vi "IMAQdx Prototyping-mod.vi"() -> ()   [LabVIEW 2017]
uses:
  <vilib>/userdefined/High Color/IMAQdx.ctl
  <vilib>/vision/Avi.llb/IMAQ AVI2 Codec Path.ctl
  <vilib>/vision/driver/IMAQdx.llb/IMAQdx Buffer Number Mode.ctl
  <vilib>/vision/driver/NI_Vision_Acquisition_Software.lvlib
  <vilib>/vision/NI_Vision_Development_Module.lvlib
panel:
  out "Missed frames!":bool
  out "Buffer Number Delta":u32
  out "Skipped Buffer Count":u32
  out "Acquired Frame Rate":dbl
  out "Processed Frame Rate":dbl
  in  "Vertical Stop Button":bool
  in  "Capture video":bool
  out "Codec Names":string[](array[string])
  out "element":string
  in  "index":i32=6
  in  "AVI Path":path=path "C:/Users/Theo/Desktop/AVI compression tests"
  in  "Resolution":dbl(slide)=1.0 step=0.1 scale=0.1..1.0
  in  "Interpolation Type":u32(ring) items=["Zero Order", "Bi-Linear", "Quadratic", "Cubic Spline"]
  out "Image 2":T1(plugin-control)
  out "ms":u32 format="%.0f ms"
  out "Image":T1(plugin-control)
  in  "Session In":T2="cam0"
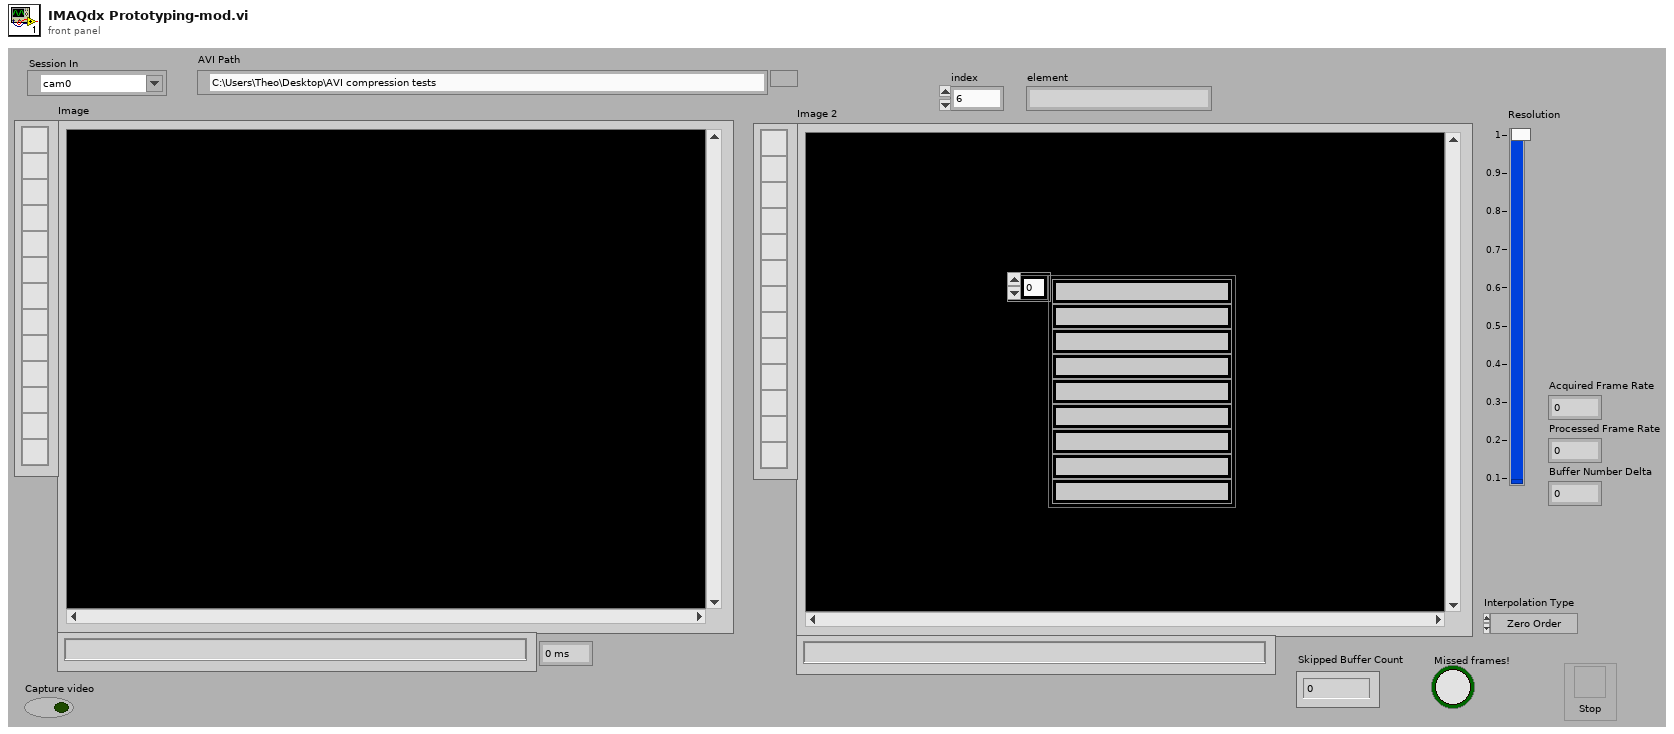
[diagram p1: front panel]
types:
  T1 = typedef "IMAQ Image.ctl" = refnum<image>
  T2 = typedef "IMAQdx.ctl" = refnum<k21>
  T3 = typedef "IMAQ AVI2 Codec Path.ctl" = u32
  T4 = typedef "Image Type" = u32
  T5 = enum16{"open", "replace", "create", "open or create", "replace or create", "replace or create with confirmation"}
  T6 = typedef "IMAQ AVI2 Refnum.ctl" = refnum<k20>
  T7 = typedef "NI_Vision_Acquisition_Software.lvlib/IMAQdx Buffer Number Mode.ctl" = enum32{"Next", "Last", "Buffer Number", "Every", "Last New"}
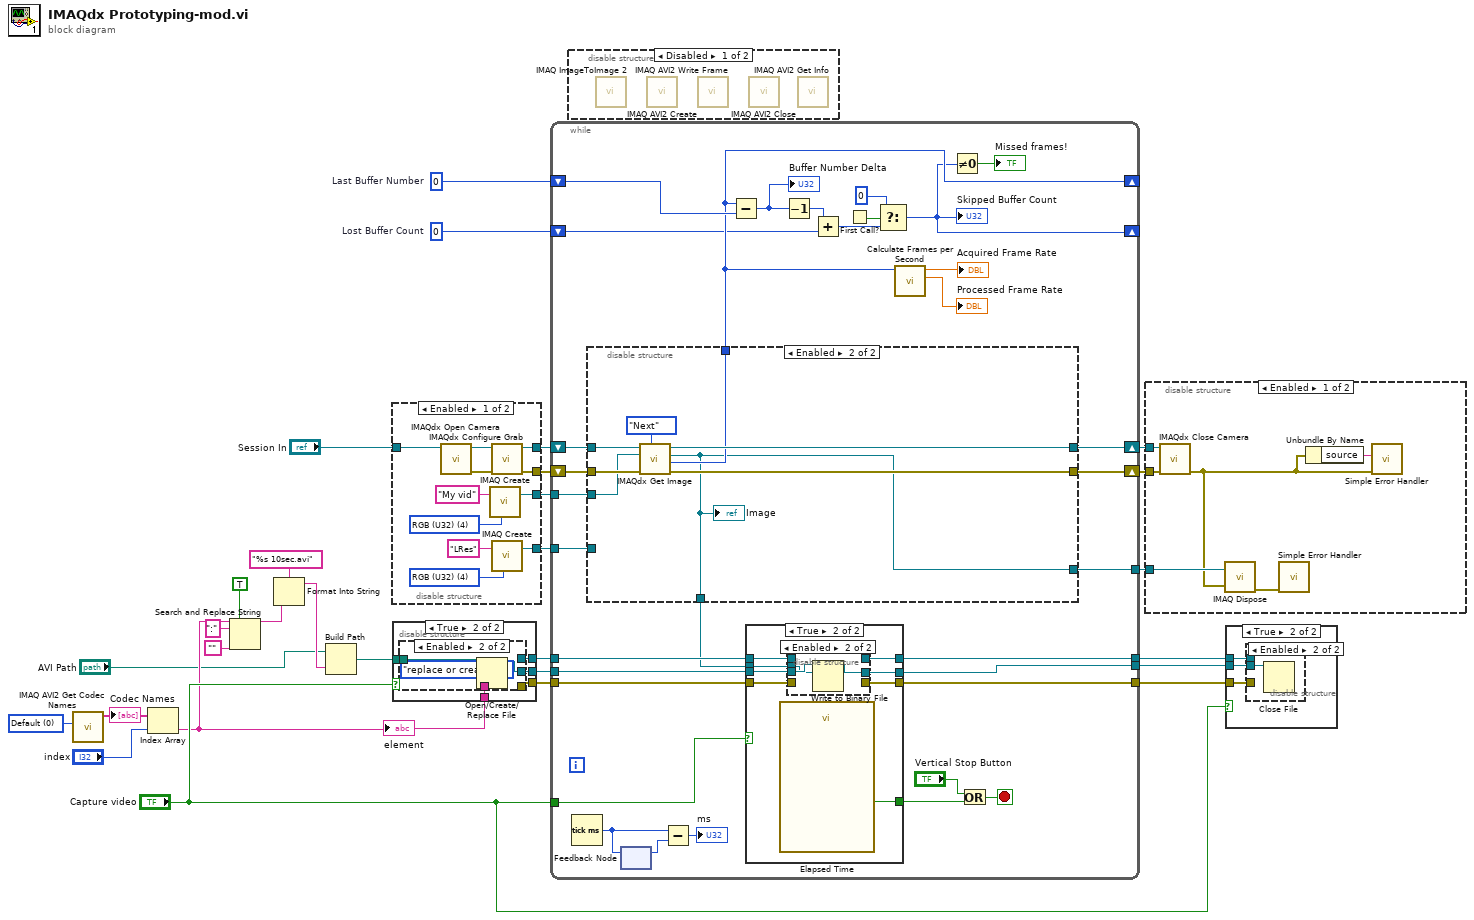
[diagram p0: block diagram]
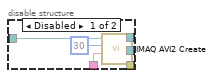
[diagram p5: hidden frame]
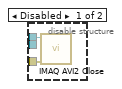
[diagram p7: hidden frame]
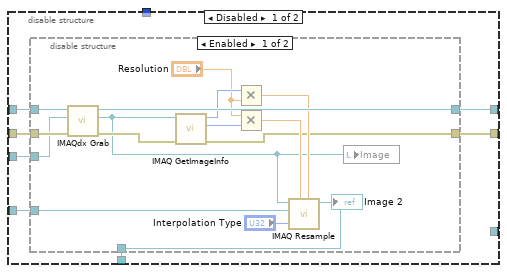
[diagram p9: hidden frame]
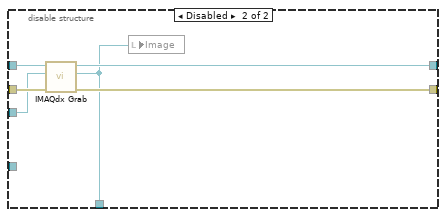
[diagram p10: hidden frame]
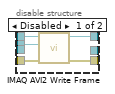
[diagram p12: hidden frame]
diagram:
  w10 = u32 0  # Lost Buffer Count
  w11 = u32 0  # Last Buffer Number
  w29 = T3 0 items=["Default", "System", "Built in Vision"] ("Codec Source")
  n1 = call "IMAQ AVI2 Get Codec Names"("Codec Source"=w29) -> ("Codec Names"=w22:string[])  [unwired: 9 in, 1 out]
  "Codec Names" <- w22
  n2 = Index Array(array=w22, index="index") -> (element=w6:string)
  "element" <- w6
  n3 = Search and Replace String(replace all?=TRUE ("replace all? (F)"), input string=w6, search string=":", replace string="" ("replace string (\"\")")) -> (result string=w7:string)  [unwired: 4 in, 3 out]
  n4 = Format Into String(format string="%s 10sec.avi", w7) -> (resulting string=w13:string)  [unwired: 2 in, 1 out]
  n5 = Build Path(base path="AVI Path", name or relative path=w13) -> (appended path=w15:path)
  n6 = disable-structure shown="Enabled" {
    disable-tunnel: [w40 _] -> w28
    disable-tunnel: [w39 _] -> w25
    disable-tunnel: [w36 _] -> w24
    disable-tunnel: [w34 _] -> w23
    disable-tunnel: "Session In" -> [w32 _]
    frame Enabled {
      w33 = T4 4 items=["Grayscale (U8)", "Grayscale (I16)", "Grayscale (SGL)", "Complex (CSG)", "RGB (U32)", "HSL (U32)", "RGB (U64)", "Grayscale (U16)"] ("Image Type")
      w37 = T4 4 items=["Grayscale (U8)", "Grayscale (I16)", "Grayscale (SGL)", "Complex (CSG)", "RGB (U32)", "HSL (U32)", "RGB (U64)", "Grayscale (U16)"] ("Image Type")
      n7 = call <vilib>:"IMAQdx Open Camera.vi"("Session In"=w32) -> ("error out"=w30:errorcluster, "Session Out"=w31:T2)  [unwired: 9 in]
      n8 = call "IMAQ Create"("Image Name"="My vid", "Image Type"=w37) -> ("New Image"=w36:T1)  [unwired: 3 in, 1 out]
      n9 = call <vilib>:"IMAQdx Configure Grab.vi"("error in"=w30, "Session In"=w31) -> ("error out"=w39:errorcluster, "Session Out"=w40:T2)  [unwired: 8 in]
      n10 = call "IMAQ Create"("Image Name"="LRes", "Image Type"=w33) -> ("New Image"=w34:T1)  [unwired: 3 in, 1 out]
    }
    frame Disabled {
    }
  }
  n11 = case shown="True" "Capture video" {
    tunnel: w15 -> [_ w45]
    tunnel: [_ w44] -> w20
    tunnel: [_ w43] -> w19
    tunnel: w6 -> [_ w42]
    tunnel: [_ w41] -> w2
    frame False {
    }
    frame True {
      n12 = disable-structure shown="Enabled" {
        disable-tunnel: w45 -> [w50 w53]
        disable-tunnel: [w48 _] -> w44
        disable-tunnel: [w47 _] -> w43
        disable-tunnel: w42 -> [w46 _]
        disable-tunnel: [_ w52] -> w41
        frame Disabled {
          n13 = call "IMAQ AVI2 Create"("Codec"=w46, "Frames Per Second"=u32 30, "AVI Path"=w50) -> ("error out"=w47:errorcluster, "AVI Refnum"=w48:T6)  [unwired: 7 in]
        }
        frame Enabled {
          n14 = Open/Create/Replace File(file path (use dialog)=w53, operation (0:open)=T5."replace or create") -> (refnum out=w52:refnum<file>)  [unwired: 4 in, 2 out]
        }
      }
    }
  }
  n15 = while {
    shift-right: [w85] -> w27
    shift-left: w28 -> [w86]
    shift-right: [w75] -> w26
    shift-left: w25 -> [w84]
    tunnel: w24 -> [w83]
    tunnel: w23 -> [w79]
    tunnel: w20 -> [w78]
    tunnel: w19 -> [w77]
    tunnel: [w76] -> w18
    tunnel: [w73] -> w17
    tunnel: "Capture video" -> [w72]
    tunnel: [w68] -> w12
    shift-right: [w59] -> _
    shift-left: w11 -> [w60]
    shift-right: [w57] -> _
    shift-left: w10 -> [w58]
    tunnel: w2 -> [w55]
    tunnel: [w54] -> w1
    stop <- w71 stop-if-true
    n16 = Tick Count (ms)() -> (millisecond timer value=w81:u32)
    n17 = disable-structure shown="Enabled" {
      disable-tunnel: w86 -> [w93 w121]
      disable-tunnel: [w92 w119] -> w85
      disable-tunnel: w84 -> [w91 w120]
      disable-tunnel: w83 -> [w90 w116]
      disable-tunnel: w79 -> [w89 _]
      disable-tunnel: [w88 w118] -> w75
      disable-tunnel: [w87 w115] -> w74
      disable-tunnel: [_ w115] -> w68
      disable-tunnel: [_ w117] -> w59
      frame Disabled {
        n18 = disable-structure shown="Enabled" {
          disable-tunnel: w93 -> [w108 w114]
          disable-tunnel: [w107 w110] -> w92
          disable-tunnel: w91 -> [w106 w113]
          disable-tunnel: w90 -> [w105 w112]
          disable-tunnel: w89 -> [w103 _]
          disable-tunnel: [w96 w111] -> w88
          disable-tunnel: [w94 w109] -> w87
          frame Enabled {
            n19 = call <vilib>:"IMAQdx Grab.vi"("error in"=w106, "Image In"=w105, "Session In"=w108) -> ("error out"=w97:errorcluster, "Image Out"=w95:T1, "Session Out"=w107:T2)  [unwired: 5 in, 1 out]
            n20 = call "IMAQ GetImageInfo"("error in (no error)"=w97, "Image"=w95) -> ("error out"=w96:errorcluster, "Y Resolution"=w101:i32, "X Resolution"=w102:i32)  [unwired: 2 in, 5 out]
            n21 = Multiply(x=w102, y="Resolution") -> (x*y=w100:dbl)
            n22 = Multiply(x="Resolution", y=w101) -> (x*y=w99:dbl)
            n23 = call "IMAQ Resample"("X Resolution"=w100, "Y Resolution"=w99, "Interpolation Type"="Interpolation Type", "Image Dst"=w103, "Image Src"=w95) -> ("Image Dst Out"=w94:T1)  [unwired: 5 in, 1 out]
            "Image 2" <- w94
            n24 = local write "Image"(w95) -> ()
          }
          frame Disabled {
            n25 = call <vilib>:"IMAQdx Grab.vi"("error in"=w113, "Image In"=w112, "Session In"=w114) -> ("error out"=w111:errorcluster, "Image Out"=w109:T1, "Session Out"=w110:T2)  [unwired: 5 in, 1 out]
            n26 = local write "Image"(w109) -> ()
          }
        }
      }
      frame Enabled {
        n27 = call <vilib>:"IMAQdx Get Image.vi"("Buffer Number Mode (Next)"=IMAQdx_Buffer_Number_Mode."Next", "error in"=w120, "Image In"=w116, "Session In"=w121) -> ("error out"=w118:errorcluster, "Buffer Number Out"=w117:u32, "Image Out"=w115:T1, "Session Out"=w119:T2)  [unwired: 1 in, 3 out]
        "Image" <- w115
      }
    }
    n28 = feedback #1() -> (w80:u32)  [unwired: 1 in]
    n29 = feedback-in #1(w81) -> ()
    n30 = Subtract(x=w81, y=w80) -> (x-y=→"ms":u32)
    n31 = Subtract(x=w59, y=w60) -> (x-y=w67:u32)
    "Buffer Number Delta" <- w67
    n32 = case shown="True" w72 {
      tunnel: w78 -> [w124 w132]
      tunnel: w77 -> [w123 w131]
      tunnel: [w124 w130] -> w76
      tunnel: w74 -> [_ w128]
      tunnel: [_ w127] -> w70
      tunnel: [w123 w129] -> w73
      tunnel: w55 -> [_ w126]
      tunnel: [_ w125] -> w54
      frame False {
      }
      frame True {
        n33 = call "Elapsed Time"() -> ("Time has Elapsed"=w127:bool)  [unwired: 12 in, 7 out]
        n34 = disable-structure shown="Enabled" {
          disable-tunnel: w132 -> [w137 _]
          disable-tunnel: w131 -> [w136 _]
          disable-tunnel: [w135 _] -> w130
          disable-tunnel: [w134 _] -> w129
          disable-tunnel: w128 -> [w133 w138]
          disable-tunnel: w126 -> [_ w140]
          disable-tunnel: [_ w139] -> w125
          frame Disabled {
            n35 = call "IMAQ AVI2 Write Frame"("error in (no error)"=w136, "Image"=w133, "AVI Refnum"=w137) -> ("error out"=w134:errorcluster, "AVI Refnum (duplicate)"=w135:T6)  [unwired: 6 in, 1 out]
          }
          frame Enabled {
            n36 = Write to Binary File(file (use dialog)=w140, data=w138) -> (refnum out=w139:refnum<file>)  [unwired: 4 in, 2 out]
          }
        }
      }
    }
    n37 = Decrement(x=w67) -> (x-1=w66:u32)
    n38 = Add(x=w66, y=w58) -> (x+y=w65:u32)
    n39 = First Call?() -> (First Call?: T/F=w64:bool)
    n40 = Select(t=u32 0, s=w64, f=w65) -> (s? t:f=w57:u32)
    "Skipped Buffer Count" <- w57
    n41 = call <vilib>:"Calculate Frames per Second.vi"("Buffer Number"=w59) -> ("Processed Frames/s"=→"Processed Frame Rate":dbl, "Acquired Frames/s"=→"Acquired Frame Rate":dbl)  [unwired: 8 in, 1 out]
    n42 = Not Equal To 0?(x=w57) -> (x != 0?=→"Missed frames!":bool)
    n43 = Or(x="Vertical Stop Button", y=w70) -> (x .or. y?=w71:bool)
  }
  n44 = disable-structure shown="Disabled" {
    frame Disabled {
      n45 = call "IMAQ ImageToImage 2"() -> ()  [unwired: 10 in, 2 out]
      n46 = call "IMAQ AVI2 Create"() -> ()  [unwired: 10 in, 2 out]
      n47 = call "IMAQ AVI2 Write Frame"() -> ()  [unwired: 9 in, 3 out]
      n48 = call "IMAQ AVI2 Close"() -> ()  [unwired: 11 in, 1 out]
      n49 = call "IMAQ AVI2 Get Info"() -> ()  [unwired: 7 in, 5 out]
    }
    frame Enabled {
    }
  }
  n50 = disable-structure shown="Enabled" {
    disable-tunnel: w27 -> [w145 _]
    disable-tunnel: w26 -> [w144 _]
    disable-tunnel: w12 -> [w142 _]
    frame Enabled {
      n51 = call <vilib>:"IMAQdx Close Camera.vi"("error in"=w144, "Session In"=w145) -> ("error out"=w141:errorcluster)  [unwired: 9 in]
      n52 = call "IMAQ Dispose"("Image"=w142, "error in (no error)"=w141) -> ("error out"=w143:errorcluster)  [unwired: 4 in]
      n53 = call <vilib>:"Simple Error Handler.vi"("error in (no error)"=w143) -> ()  [unwired: 1 in, 8 out]
      n54 = Unbundle By Name(w141) -> ("source"=w146:string)
      n55 = call <vilib>:"Simple Error Handler.vi"("error source (\" \")"=w146, "error in (no error)"=w141) -> ()  [unwired: 3 in, 5 out]
    }
    frame Disabled {
    }
  }
  n56 = case shown="True" "Capture video" {
    tunnel: w18 -> [_ w149]
    tunnel: w17 -> [_ w148]
    tunnel: w1 -> [_ w147]
    frame False {
    }
    frame True {
      n57 = disable-structure shown="Enabled" {
        disable-tunnel: w149 -> [w151 _]
        disable-tunnel: w148 -> [w150 _]
        disable-tunnel: w147 -> [_ w152]
        frame Disabled {
          n58 = call "IMAQ AVI2 Close"("error in (no error)"=w150, "AVI Refnum"=w151) -> ()  [unwired: 9 in, 1 out]
        }
        frame Enabled {
          n59 = Close File(refnum=w152) -> ()  [unwired: 1 in, 2 out]
        }
      }
    }
  }
